vi "Read Elevator Constants.vi"(8 "error in (no error)":errorcluster, 11 "Elevator in":refnum<class "Elevator.lvclass">) -> (0 "error out":errorcluster, 2 "Elevator Constants":T1, 3 "Elevator out":refnum<class "Elevator.lvclass">)   [LabVIEW 2018, in "Elevator.lvlib" / "Elevator.lvclass"]
uses:
  Elevator.lvclass
  Controls/Elevator Constants.ctl
  Elevator.lvclass/Elevator.ctl
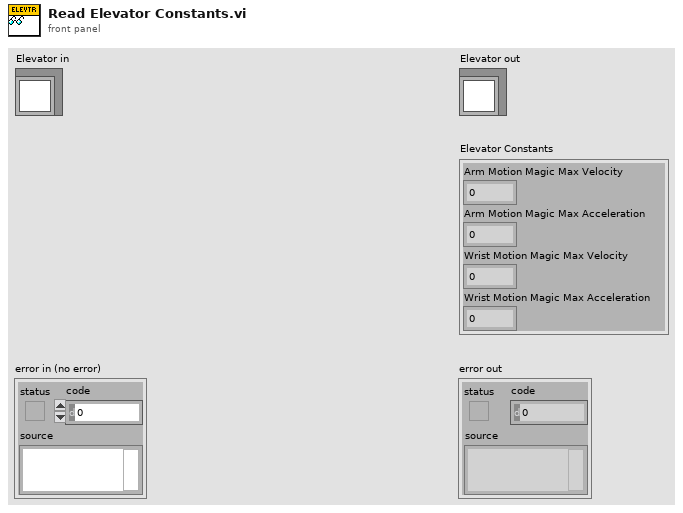
[diagram p1: front panel]
types:
  T1 = typedef "Elevator.lvlib/Elevator.lvclass/Elevator Constants.ctl" = cluster{"Arm Motion Magic Max Velocity":u32, "Arm Motion Magic Max Acceleration":u32, "Wrist Motion Magic Max Velocity":u32, "Wrist Motion Magic Max Acceleration":u32}
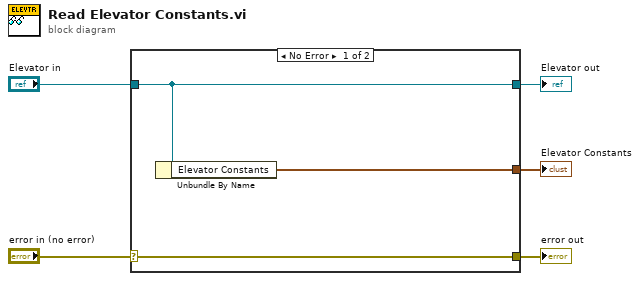
[diagram p0: block diagram]
diagram:
  n1 = case shown="No Error" "error in (no error)" {
    selector: "error in (no error)" -> [w8 w9]
    tunnel: [w8 w9] -> w4
    tunnel: [w7 w10] -> w2
    tunnel: "Elevator in" -> [w7 w10]
    tunnel: [w6 _] -> w1
    frame No Error {
      n2 = Unbundle By Name(w7) -> ("Elevator Constants"=w6:T1)
    }
    frame Error {
    }
  }
  "error out" <- w4
  "Elevator out" <- w2
  "Elevator Constants" <- w1
